vi "Dashboard-Cory.vi"(0 "DashboardData":T1) -> ()   [LabVIEW 2015]
uses:
  Typedefs/Data to Dashboard.ctl
  Typedefs/CollectorLiftStates.ctl
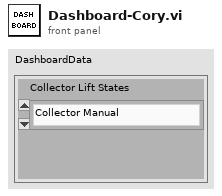
[diagram p1: front panel]
types:
  T1 = typedef "Data to Dashboard.ctl" = cluster{"Collector Lift States":T2}
  T2 = typedef "CollectorLiftStates.ctl" = enum16{"Collector Manual", "Stow", "Collect Position", "Spit Position", "Portcullis Set Up", "Portcullis Lift Up", "CDF Set Up", "Push CDF Down"}
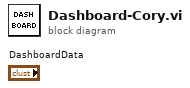
[diagram p0: block diagram]
diagram:
